vi "S2C_ExeScriptShowResult.vi"(8 "Error In":errorcluster, 11 "Result In":string) -> (0 "Error Out":errorcluster)   [LabVIEW 2015]
doc: "Shows the overall test execution results."
panel:
  out "Init":bool
  out "TestResult":string
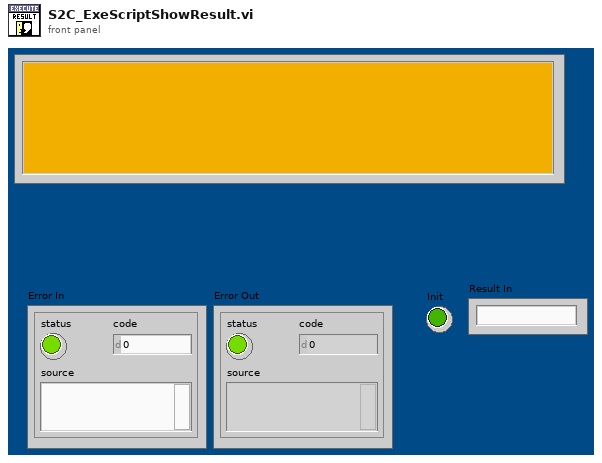
[diagram p1: front panel]
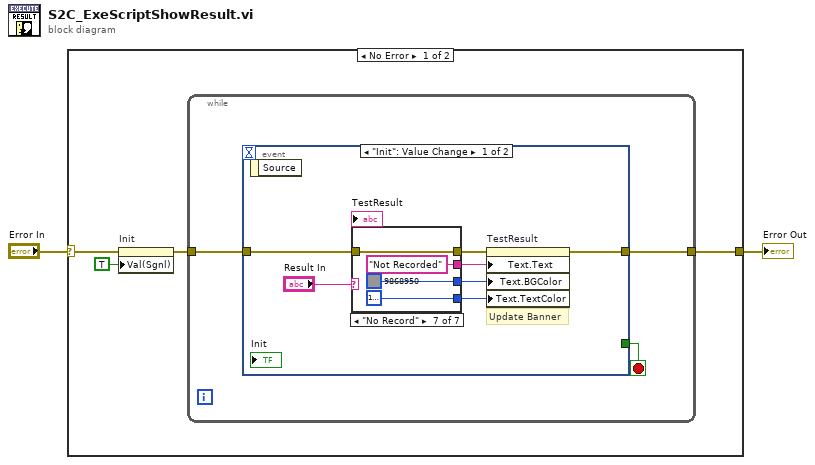
[diagram p0: block diagram]
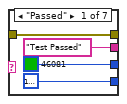
[diagram p2: hidden frame]
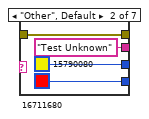
[diagram p3: hidden frame]
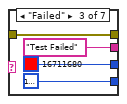
[diagram p4: hidden frame]
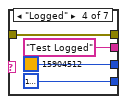
[diagram p5: hidden frame]
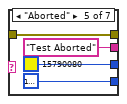
[diagram p6: hidden frame]
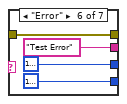
[diagram p7: hidden frame]
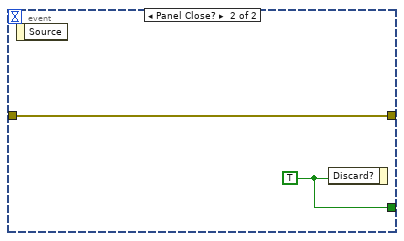
[diagram p8: hidden frame]
diagram:
  n1 = case shown="No Error" "Error In" {
    selector: "Error In" -> [w5 w47]
    tunnel: [w6 w47] -> w1
    frame No Error {
      n2 = property on="Init" class="Bool (strict)"(error in=w5, "Val(Sgnl)"=TRUE ("Value (Signaling)")) -> (error out=w4:errorcluster)  [unwired: 1 in, 1 out]
      n3 = while {
        tunnel: w4 -> [w9]
        tunnel: [w8] -> w6
        stop <- w7 stop-if-true
        n4 = event shown="[0] \"Init\": Value Change" {
          selector: _ -> [_ _]
          dyn-events: _ -> [_ _]
          timeout: _ -> [_ _]
          tunnel: w9 -> [w12 w46]
          tunnel: [w16 w46] -> w8
          tunnel: [_ w45] -> w7
          event "Init": Value Change {
            # "Update Banner"
            n5 = event-data() -> ()  [unwired: 1 in, 1 out]
            n6 = case shown="\"No Record\"" "Result In" {
              tunnel: [u32 46081 u32 15790080 u32 16711680 u32 15904512 u32 15790080 u32 16777222 u32 9868950] -> w14
              tunnel: [u32 16777226 u32 16711680 u32 16777226 u32 16777226 u32 16777222 u32 16777226 u32 16777226] -> w15
              tunnel: ["Test Passed" "Test Unknown" "Test Failed" "Test Logged" "Test Aborted" "Test Error" "Not Recorded"] -> w13
              tunnel: w12 -> [w17 w21 w25 w29 w33 w37 w41]
              tunnel: [w17 w21 w25 w29 w33 w37 w41] -> w11
              frame "Passed" {
              }
              frame "Other", Default {
              }
              frame "Failed" {
              }
              frame "Logged" {
              }
              frame "Aborted" {
              }
              frame "Error" {
              }
              frame "No Record" {
              }
            }
            n7 = property on="TestResult" class="Str"(error in=w11, "Text.Text"=w13, "Text.BGColor"=w14, "Text.TextColor"=w15) -> (error out=w16:errorcluster)  [unwired: 1 in, 1 out]
          }
          event Panel Close? {
            w45 = TRUE ("Discard?")
            n8 = event-data() -> ()  [unwired: 1 in, 1 out]
            n9 = event-data("Discard?"=w45) -> ()  [unwired: 1 in, 1 out]
          }
        }
      }
    }
    frame Error {
    }
  }
  "Error Out" <- w1
